vi "load_manual_actions.vi"(8 "error in (no error)":errorcluster, 11 "recipe_in":variant) -> (0 "error out":errorcluster, 2 "replaced_step":bool, 3 "recipe_out":variant)   [LabVIEW 2015, in "example_01.lvlib"]
uses:
  example_01.lvlib
  lv-recipe-machine/public/_controls/step.ctl
  _controls/manual_actions.ctl
  lv-recipe-machine/lv-recipe-machine.lvlib
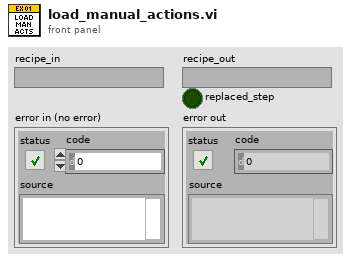
[diagram p1: front panel]
types:
  T1 = typedef "example_01.lvlib/manual_actions.ctl" = enum16{"<manual_action>", "manual_test_random", "manual_test_comparison", "manual_test_wait", "<null>"}
  T2 = typedef "lv-recipe-machine.lvlib/step.ctl" = cluster{"name":string, "data":variant, "step_vi_reference":refnum<vi>}
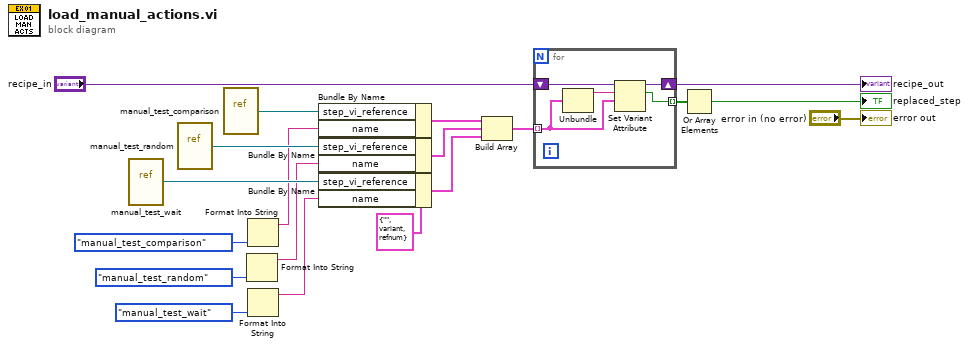
[diagram p0: block diagram]
diagram:
  w9 = T2 {"name"="", "data"=variant, "step_vi_reference"=refnum} ("step")
  n1 = vi-ref "manual_test_wait.vi"() -> (w19:refnum<vi>)
  n2 = vi-ref "manual_test_random.vi"() -> (w18:refnum<vi>)
  n3 = vi-ref "manual_test_comparison.vi"() -> (w17:refnum<vi>)
  n4 = Format Into String(manual_actions."manual_test_random" ("action")) -> (resulting string=w15:string)  [unwired: 3 in, 1 out]
  n5 = Format Into String(manual_actions."manual_test_comparison" ("action")) -> (resulting string=w16:string)  [unwired: 3 in, 1 out]
  n6 = Format Into String(manual_actions."manual_test_wait" ("action")) -> (resulting string=w14:string)  [unwired: 3 in, 1 out]
  n7 = Bundle By Name(cluster=w9, "step_vi_reference"=w17, "name"=w16) -> (w5:T2)
  n8 = Bundle By Name(cluster=w9, "step_vi_reference"=w18, "name"=w15) -> (w6:T2)
  n9 = Bundle By Name(cluster=w9, "step_vi_reference"=w19, "name"=w14) -> (w10:T2)
  n10 = Build Array(w5, w6, w10) -> (w7:T2[])
  n11 = for {
    tunnel: w7 -> [w22] mode=indexing
    shift-right: [w23] -> w8
    shift-left: "recipe_in" -> [w24]
    tunnel: [w20] -> w2 mode=indexing
    n12 = Unbundle(w22) -> ("name"=w21:string)  [unwired: 2 out]
    n13 = Set Variant Attribute(Variant=w24, name=w21, value=w22) -> (Variant out=w23:variant, replaced=w20:bool)  [unwired: 1 in, 1 out]
  }
  "recipe_out" <- w8
  n14 = Or Array Elements(Boolean array=w2) -> (logical OR=→"replaced_step":bool)
  "error out" <- "error in (no error)"
